vi "Get VI Connector Pane image and Description.vi"(8 "error in":errorcluster, 11 "VI in":refnum<vi>) -> (0 "error out":errorcluster, 1 "VI Description":string, 2 "VI Connector Pane":picture, 3 "Vi out":refnum<vi>)   [LabVIEW 2020, in "Panter Dashboard.lvlib"]
doc: "Get the connector pane of the vi by getting it's reference"
uses:
  Panter Dashboard.lvlib
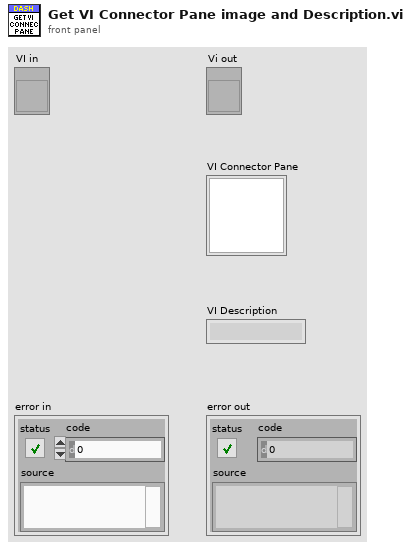
[diagram p1: front panel]
types:
  T1 = typedef "imagedata.ctl" = cluster{"image type":i32, "image depth":i32, "image":u8[], "mask":u8[], "colors":u32[], "Rectangle":cluster{"left":i16, "top":i16, "right":i16, "bottom":i16}}
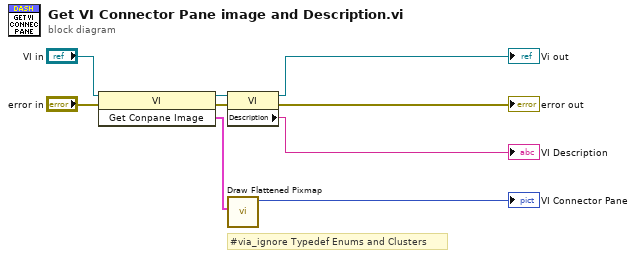
[diagram p0: block diagram]
diagram:
  # "#via_ignore Typedef Enums and Clusters"
  n1 = invoke class="VI" method="Get Conpane Image"(reference="VI in", error in="error in") -> (reference out=w6:refnum<vi>, error out=w9:errorcluster, "Get Conpane Image"=w4:T1)  [unwired: 1 in]
  n2 = property class="VI"(reference=w6, error in=w9) -> (reference out=→"Vi out":refnum<vi>, error out=→"error out":errorcluster, "Description"=→"VI Description":string)
  n3 = call <vilib>:"Draw Flattened Pixmap.vi"("image data"=w4) -> ("new picture"=→"VI Connector Pane":picture)  [unwired: 8 in]
